vi "get FPGA Resource Info.vi"(8 "error in (no error)":errorcluster, 11 "CD Ref in":T1 format="%.0x") -> (0 "error out":errorcluster, 2 "Value":variant, 3 "Item Ref out":T1 format="%.0x")   [LabVIEW 2016, in "FPGA RM Shared API.lvlib"]
uses:
  FPGA RM Shared API.lvlib
  <vilib>/NI Veristand/Custom Device API/Custom Device Item Ref.ctl
  <vilib>/NI Veristand/Custom Device API/Get Item Property (Variant).vi
  <vilib>/NI VeriStand/Custom Device API/Custom Device API.lvlib
  System Definition/FPGA RM System Definition API.lvlib
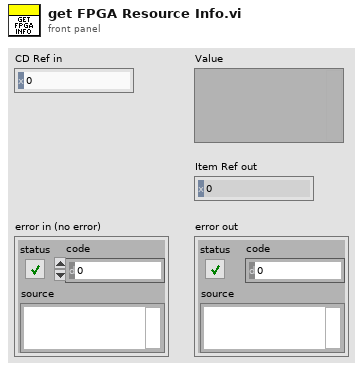
[diagram p1: front panel]
types:
  T1 = typedef "Custom Device API.lvlib/Custom Device Item Ref.ctl" = u64
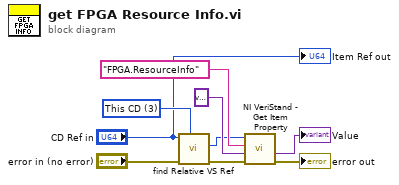
[diagram p0: block diagram]
diagram:
  w5 = u16 3 items=["Targets", "Controller", "Custom Devices", "This CD", "This CD/Group", "This CD/Group/SubGroup"] ("Relative Type")
  n1 = call "find Relative VS Ref.vi"("Relative Type"=w5, "error in (no error)"="error in (no error)", "Item Ref in"="CD Ref in") -> ("error out"=w1:errorcluster, "Relative Item Ref Out"=w2:T1)  [unwired: 4 in, 3 out]
  n2 = call-poly <vilib>:"NI VeriStand - Get Item Property.vi"("error in (no error)"=w1, "Default Value"=variant ("Variant"), "Property Name"="FPGA.ResourceInfo", "Item Ref in"=w2) -> ("error out"=→"error out":errorcluster, "Value"=→"Value":variant)  [unwired: 4 in, 2 out]
  "Item Ref out" <- "CD Ref in"
